vi "Remove From Grouped Segments.vi"(5 "Index":i32, 7 "Length":i32, 11 "Length Grouped Segments In":cluster{cluster{i32[]}[]}[](array[cluster])) -> (3 "Length Grouped Segments":cluster{cluster{i32[]}[]}[](array[cluster]))   [LabVIEW 2020]
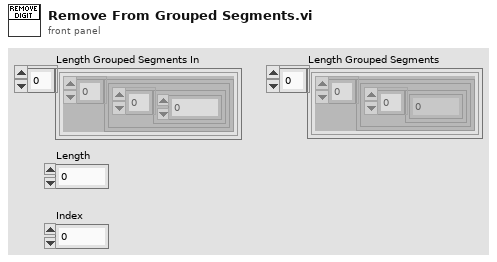
[diagram p1: front panel]
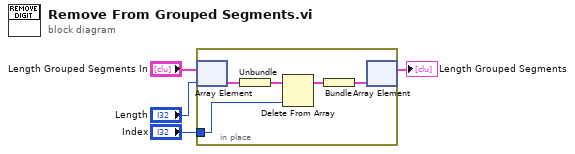
[diagram p0: block diagram]
diagram:
  n1 = in-place {
    in-place-border: "Index" -> [w7]
    n2 = in-place-array #1("Length Grouped Segments In", "Length") -> (w9:cluster{cluster{i32[]}[]})
    n3 = Unbundle(w9) -> (w8:cluster{i32[]}[])
    n4 = Delete From Array(array=w8, index=w7) -> (array with subset deleted=w6:cluster{i32[]}[])  [unwired: 1 in, 1 out]
    n5 = Bundle(w6) -> (w5:cluster{cluster{i32[]}[]})  [unwired: 1 in]
    n6 = in-place-array #1(w5) -> (→"Length Grouped Segments":cluster{cluster{i32[]}[]}[])  [unwired: 1 out]
  }
